vi "Main.vi"() -> ()   [LabVIEW 2022 SP3]
doc: "This template is for the Queued Message Handler design pattern.\n\nThe Event Handling Loop generates messages based on user interface actions.\n\nThe Message Handling Loop processes messages generated by the Event Handling Loop, or by other messages. The messages are string values, so new messages can be added easily to the Message Cases case structure in the Message Handling Loop. Each message cluster can also provide an optional value for Message Data, which is a variant that can be converted to whatever message-specific data is required."
uses:
  controls/UI Data.ctl
  support/Boiler System Globals.vi
  support/Message Queue/Message Queue.lvlib
  support/User Event - Stop/User Event - Stop.lvlib
  Boiler/Boiler.lvlib
panel:
  out "Display <Replace Me>":string
  in  "Do Something Else <Replace Me>":bool
  in  "Do Something <Replace Me>":bool
  in  "Stop Button":bool
  # "These controls have associated \"Value Changed\" events configured in the Event Structure on the diagram.\n\nReplace them (and reconfigure the Event Structure) with the controls you need for your application."
  # "This template is for the Queued Message Handler design pattern.\n\nSee the block diagram for more information on how to use this template."
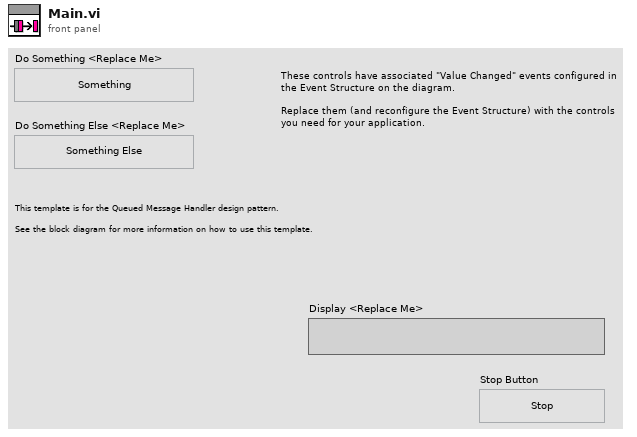
[diagram p1: front panel]
types:
  T1 = typedef "UI Data.ctl" = cluster{"Boolean <Replace Me>":bool, "String <Replace Me>":string, "Numeric <Replace Me>":dbl, "Do Something Ref":refnum<vi>, "Do Something Else Ref":refnum<vi>, "Data Display Ref":refnum<vi>, "Stop Button Ref":refnum<vi>}
  T2 = typedef "Notifiers.ctl" = cluster{"Handshake":refnum<notifier>, "Flame Level":refnum<notifier>, "Controller Exit":refnum<notifier>, "Boiler Ext":refnum<notifier>}
  T3 = typedef "Message Queue.lvlib/All Message Queues.ctl" = cluster{"MHL":refnum<queue>, "Boiler Controller":refnum<queue>, "Boiler":refnum<queue>}
  T4 = enum32{"invalid app kind", "Development System", "Run Time System", "Student Edition", "Embedded LabVIEW", "Evaluation", "Custom"}
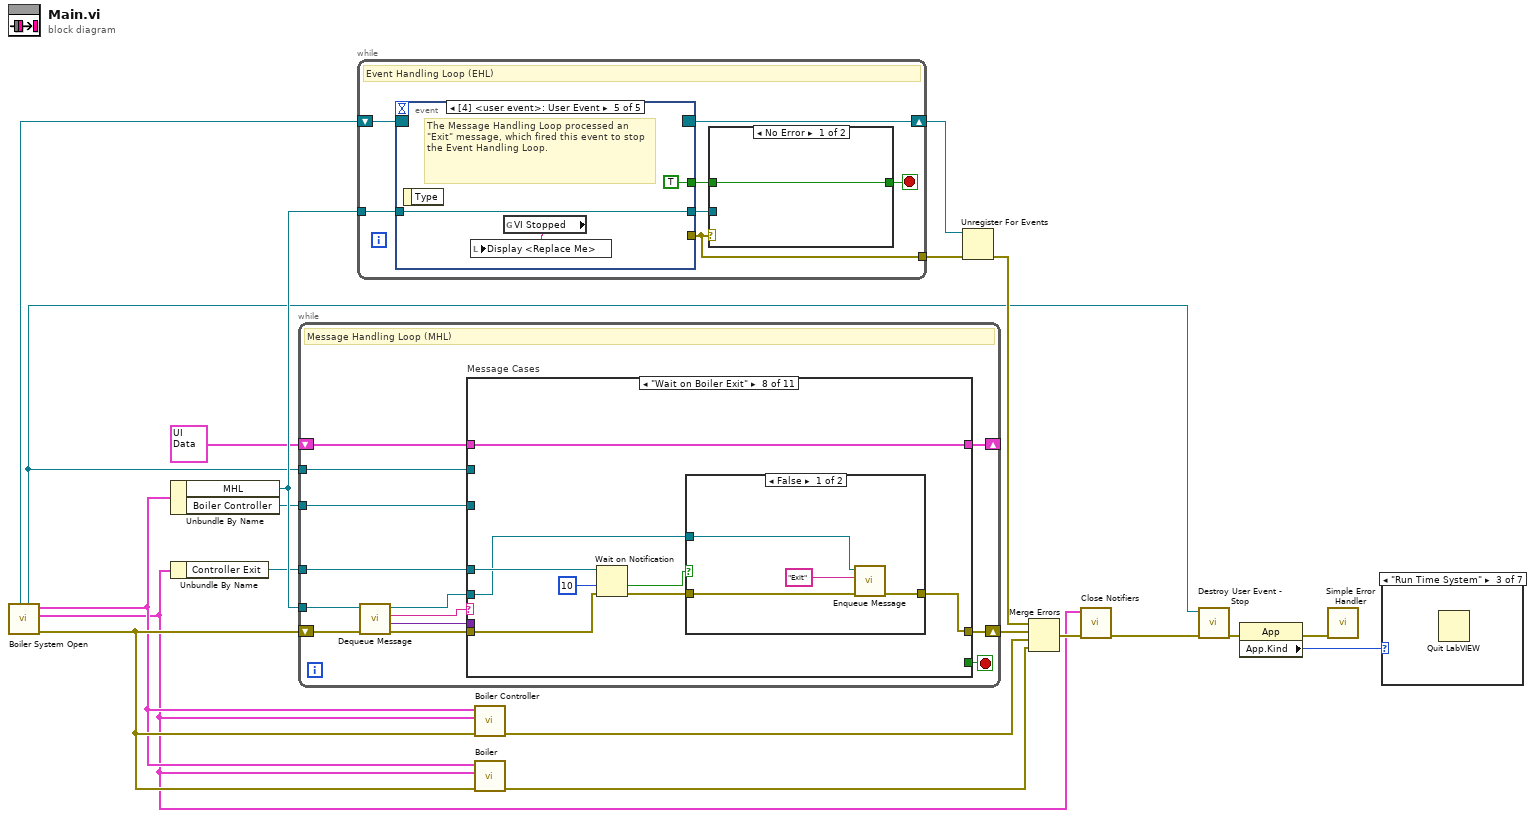
[diagram p0: block diagram]
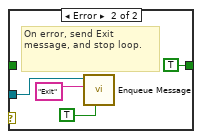
[diagram p8: hidden frame]
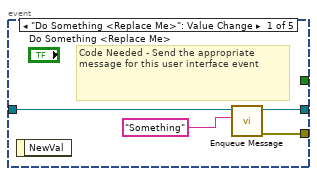
[diagram p9: hidden frame]
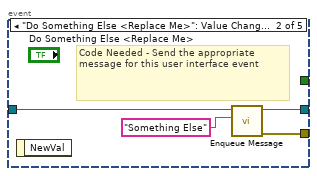
[diagram p10: hidden frame]
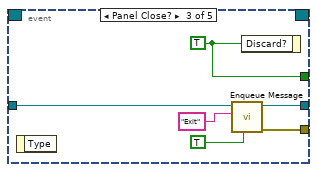
[diagram p11: hidden frame]
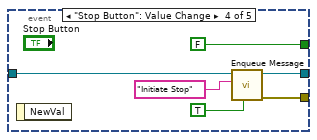
[diagram p12: hidden frame]
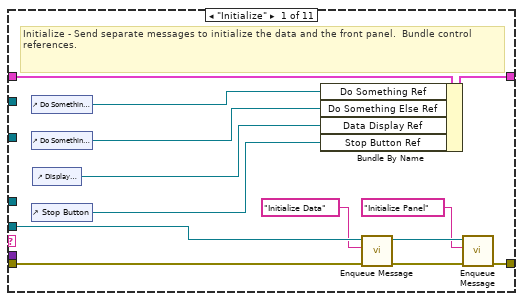
[diagram p13: hidden frame]
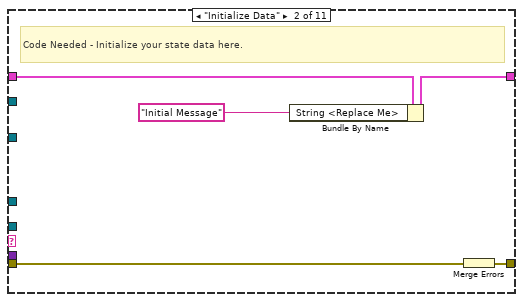
[diagram p14: hidden frame]
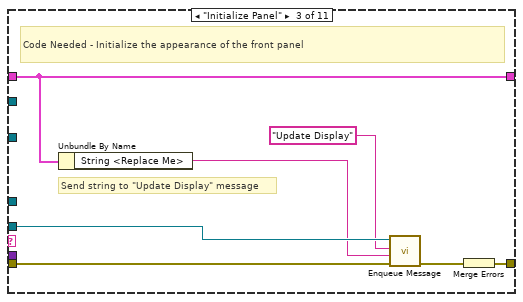
[diagram p15: hidden frame]
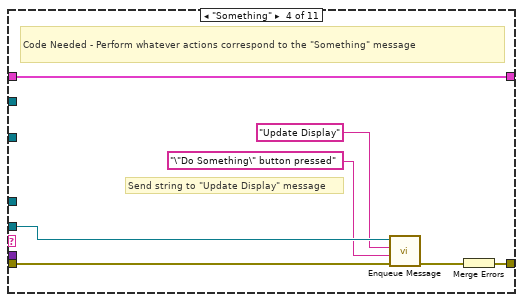
[diagram p16: hidden frame]
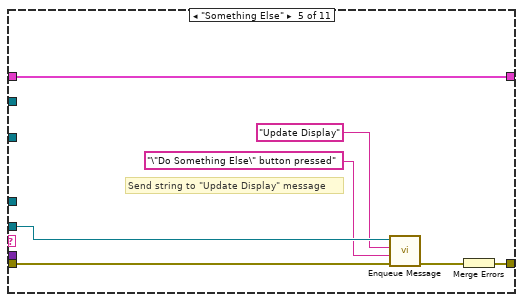
[diagram p17: hidden frame]
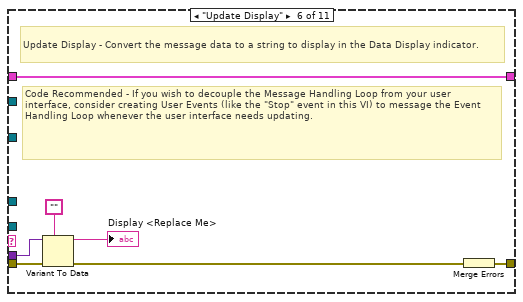
[diagram p18: hidden frame]
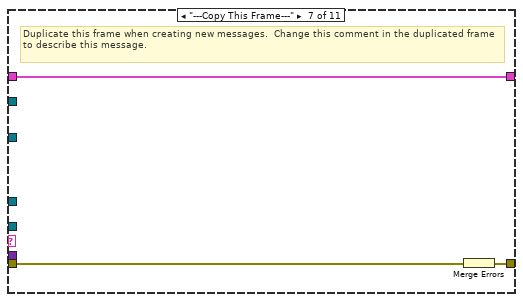
[diagram p19: hidden frame]
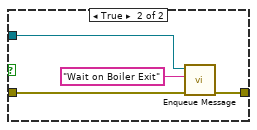
[diagram p20: hidden frame]
diagram:
  n1 = call "Boiler System Open.vi"() -> ("error out"=w7:errorcluster, "Notifiers"=w2:T2, "Message Queues"=w6:T3, "User Event - Stop"=w8:refnum<user-event>, "Stop Event Registration Refnum"=w9:refnum<event-registration>)  [unwired: 7 in]
  n2 = Unbundle By Name(w6) -> ("MHL"=w19:refnum<queue>, "Boiler Controller"=w14:refnum<queue>)
  n3 = Unbundle By Name(w2) -> ("Controller Exit"=w5:refnum<notifier>)
  n4 = while {
    tunnel: w19 -> [w23]
    shift-right: [w32] -> _
    shift-left: T1 {"Boolean <Replace Me>"=TRUE, "String <Replace Me>"="", "Numeric <Replace Me>"=0.0, "Do Something Ref"=refnum, "Do Something Else Ref"=refnum, "Data Display Ref"=refnum, "Stop Button Ref"=refnum} ("Data Cluster") -> [w33]
    tunnel: w8 -> [w29]
    shift-right: [w30] -> w20
    shift-left: w7 -> [w28]
    tunnel: w14 -> [w22]
    tunnel: w5 -> [w21]
    stop <- w31 stop-if-true
    # "Message Handling Loop (MHL)"
    n5 = call "Dequeue Message.vi"("error in"=w28, "Message Queue"=w23) -> ("error out"=w27:errorcluster, "Message Data"=w25:variant, "Message"=w26:string, "dup Message Queue"=w24:refnum<queue>)  [unwired: 6 in]
    n6 = case "Message Cases" shown="\"Wait on Boiler Exit\"" w26 {
      selector: w26 -> [_ _ _ _ _ _ _ _ _ _ w118]
      tunnel: w24 -> [w42 _ w55 w61 w68 _ _ w84 w100 w114 _]
      tunnel: w27 -> [w45 w51 w56 w63 w70 w77 w82 w89 w105 w109 _]
      tunnel: [w46 w47 w57 w64 w71 w78 w80 w83 w103 w110 w116] -> w30
      tunnel: w33 -> [w39 w50 w58 w65 w72 w79 w81 w90 w106 w113 w120]
      tunnel: [w38 w49 w58 w65 w72 w79 w81 w90 w106 w113 w120] -> w32
      tunnel: [_ _ _ _ _ _ _ _ _ TRUE _] -> w31
      tunnel: w25 -> [_ _ _ _ _ w76 _ _ _ _ _]
      tunnel: w29 -> [_ _ _ _ _ _ _ _ _ w108 _]
      tunnel: w22 -> [_ _ _ _ _ _ _ _ w99 _ _]
      tunnel: w21 -> [_ _ _ _ _ _ _ w88 _ _ _]
      frame "Initialize" {
        # "Initialize - Send separate messages to initialize the data and the front panel.  Bundle control references."
        n7 = control-ref of="Do Something <Replace Me>"() -> (w37:refnum<vi>)
        n8 = control-ref of="Do Something Else <Replace Me>"() -> (w36:refnum<vi>)
        n9 = control-ref of="Stop Button"() -> (w34:refnum<vi>)
        n10 = control-ref of="Display <Replace Me>"() -> (w35:refnum<vi>)
        n11 = Bundle By Name(cluster=w39, "Do Something Ref"=w37, "Do Something Else Ref"=w36, "Data Display Ref"=w35, "Stop Button Ref"=w34) -> (w38:T1)
        n12 = call "Enqueue Message.vi"("error in"=w45, "Message"="Initialize Data", "Message Queue"=w42) -> ("error out"=w44:errorcluster, "dup Message Queue"=w43:refnum<queue>)  [unwired: 7 in]
        n13 = call "Enqueue Message.vi"("error in"=w44, "Message"="Initialize Panel", "Message Queue"=w43) -> ("error out"=w46:errorcluster)  [unwired: 7 in, 1 out]
      }
      frame "Initialize Data" {
        # "Code Needed - Initialize your state data here."
        n14 = Bundle By Name(cluster=w50, "String <Replace Me>"="Initial Message" ("Initial Message")) -> (w49:T1)
        n15 = Merge Errors(w51) -> (w47:errorcluster)
      }
      frame "Initialize Panel" {
        # "Send string to \"Update Display\" message"
        # "Code Needed - Initialize the appearance of the front panel"
        n16 = Unbundle By Name(w58) -> ("String <Replace Me>"=w52:string)
        n17 = call "Enqueue Message.vi"("error in"=w56, "Message Data"=w52, "Message"="Update Display", "Message Queue"=w55) -> ("error out"=w54:errorcluster)  [unwired: 6 in, 1 out]
        n18 = Merge Errors(w54) -> (w57:errorcluster)
      }
      frame "Something" {
        # "Send string to \"Update Display\" message"
        # "Code Needed - Perform whatever actions correspond to the \"Something\" message"
        n19 = call "Enqueue Message.vi"("error in"=w63, "Message Data"="\"Do Something\" button pressed" ("\"Do Something\" button pressed"), "Message"="Update Display", "Message Queue"=w61) -> ("error out"=w62:errorcluster)  [unwired: 6 in, 1 out]
        n20 = Merge Errors(w62) -> (w64:errorcluster)
      }
      frame "Something Else" {
        # "Send string to \"Update Display\" message"
        n21 = call "Enqueue Message.vi"("error in"=w70, "Message Data"="\"Do Something Else\" button pressed" ("\"Do Something Else\" button pressed"), "Message"="Update Display", "Message Queue"=w68) -> ("error out"=w69:errorcluster)  [unwired: 6 in, 1 out]
        n22 = Merge Errors(w69) -> (w71:errorcluster)
      }
      frame "Update Display" {
        # "Code Recommended - If you wish to decouple the Message Handling Loop from your user interface, consider creating User Events (like the \"Stop\" event in this VI) to message the Event Handling Loop whenever the user interface needs updating."
        # "Update Display - Convert the message data to a string to display in the Data Display indicator."
        n23 = Variant To Data(error in=w77, type="", Variant=w76) -> (data=→"Display <Replace Me>":string, error out=w74:errorcluster)
        n24 = Merge Errors(w74) -> (w78:errorcluster)
      }
      frame "---Copy This Frame---" {
        # "Duplicate this frame when creating new messages.  Change this comment in the duplicated frame to describe this message."
        n25 = Merge Errors(w82) -> (w80:errorcluster)
      }
      frame "Wait on Boiler Exit" {
        n26 = Wait on Notification(notifier=w88, timeout in ms (-1)=10, error in (no error)=w89) -> (timed out?=w85:bool, error out=w86:errorcluster)  [unwired: 1 in, 2 out]
        n27 = case shown="False" w85 {
          tunnel: w86 -> [w93 w98]
          tunnel: w84 -> [w92 w97]
          tunnel: [w94 w96] -> w83
          frame False {
            n28 = call "Enqueue Message.vi"("error in"=w93, "Message"="Exit", "Message Queue"=w92) -> ("error out"=w94:errorcluster)  [unwired: 7 in, 1 out]
          }
          frame True {
            n29 = call "Enqueue Message.vi"("error in"=w98, "Message"="Wait on Boiler Exit", "Message Queue"=w97) -> ("error out"=w96:errorcluster)  [unwired: 7 in, 1 out]
          }
        }
      }
      frame "Initiate Stop" {
        # "When stopping, first send a message to stop the boiler controller.\nThen wait for the boiler and boiler controller to ext"
        n30 = call "Enqueue Message.vi"("error in"=w105, "Message"="Exit", "Message Queue"=w99) -> ("error out"=w104:errorcluster)  [unwired: 7 in, 1 out]
        n31 = call "Enqueue Message.vi"("error in"=w104, "Message"="Wait on Boiler Exit", "Message Queue"=w100) -> ("error out"=w103:errorcluster)  [unwired: 7 in, 1 out]
      }
      frame "Exit" {
        # "Stop the VI"
        # "Release the message queue reference"
        n32 = call "Fire User Event - Stop.vi"("User Event - Stop"=w108) -> ("error out"=w107:errorcluster)  [unwired: 10 in]
        n33 = Release Queue(queue=w114, error in (no error)=w109) -> (error out=w111:errorcluster)  [unwired: 1 in, 2 out]
        n34 = Merge Errors(w107, w111) -> (w110:errorcluster)
      }
      frame Default {
        # "'Default' case only runs if there is a message that isn't defined in any of the other cases.  Output a programming error."
        n35 = Format Into String(format string="The invalid message string \"%s\" was received in the Message Handling Loop." ("Unknown Message Error Text"), w118) -> (resulting string=w115:string)  [unwired: 2 in, 1 out]
        n36 = call <vilib>:"Error Cluster From Error Code.vi"("error message (\"\")"=w115, "error code (0)"=1) -> ("error out"=w116:errorcluster)  [unwired: 7 in]
      }
    }
  }
  n37 = while {
    tunnel: w19 -> [w127]
    tunnel: [w123] -> w17
    shift-right: [w121] -> w16
    shift-left: w9 -> [w122]
    stop <- w125 stop-if-true
    # "Event Handling Loop (EHL)"
    n38 = event shown="[4] <user event>: User Event" {
      selector: w122 -> [_ _ _ _ _]
      dyn-events: [_ _ _ _ _] -> w121
      timeout: _ -> [_ _ _ _ _]
      tunnel: [_ _ w146 FALSE ("Discard?") TRUE ("Discard?")] -> w126
      tunnel: w127 -> [w136 w140 w145 w152 w155]
      tunnel: [w135 w138 w144 w151 _] -> w123
      tunnel: [w134 w139 w143 w149 w155] -> w124
      event "Do Something <Replace Me>": Value Change {
        # "Code Needed - Send the appropriate message for this user interface event"
        n39 = event-data() -> ()  [unwired: 1 in, 1 out]
        n40 = call "Enqueue Message.vi"("Message"="Something", "Message Queue"=w136) -> ("error out"=w135:errorcluster, "dup Message Queue"=w134:refnum<queue>)  [unwired: 8 in]
      }
      event "Do Something Else <Replace Me>": Value Change {
        # "Code Needed - Send the appropriate message for this user interface event"
        n41 = event-data() -> ()  [unwired: 1 in, 1 out]
        n42 = call "Enqueue Message.vi"("Message"="Something Else", "Message Queue"=w140) -> ("error out"=w138:errorcluster, "dup Message Queue"=w139:refnum<queue>)  [unwired: 8 in]
      }
      event Panel Close? {
        w146 = TRUE ("Discard?")
        n43 = event-data() -> ()  [unwired: 1 in, 1 out]
        n44 = call "Enqueue Message.vi"("Priority Message? (F)"=TRUE, "Message"="Exit", "Message Queue"=w145) -> ("error out"=w144:errorcluster, "dup Message Queue"=w143:refnum<queue>)  [unwired: 7 in]
        n45 = event-data("Discard?"=w146) -> ()  [unwired: 1 in, 1 out]
      }
      event "Stop Button": Value Change {
        n46 = event-data() -> ()  [unwired: 1 in, 1 out]
        n47 = call "Enqueue Message.vi"("Priority Message? (F)"=TRUE, "Message"="Initiate Stop", "Message Queue"=w152) -> ("error out"=w151:errorcluster, "dup Message Queue"=w149:refnum<queue>)  [unwired: 7 in]
      }
      event User Event {
        # "The Message Handling Loop processed an \"Exit\" message, which fired this event to stop the Event Handling Loop."
        n48 = event-data() -> ()  [unwired: 1 in, 1 out]
        n49 = global read "Boiler System Globals.vi" "VI Stopped"() -> (w153:string)
        n50 = local write "Display <Replace Me>"(w153) -> ()
      }
    }
    n51 = case shown="No Error" w123 {
      tunnel: [w128 TRUE ("Discard?")] -> w125
      tunnel: w126 -> [w128 _]
      tunnel: w124 -> [_ w131]
      frame No Error {
      }
      frame Error {
        # "On error, send Exit message, and stop loop."
        n52 = call "Enqueue Message.vi"("Priority Message? (F)"=TRUE, "Message"="Exit", "Message Queue"=w131) -> ()  [unwired: 7 in, 2 out]
      }
    }
  }
  n53 = call "Boiler Controller.vi"("error in"=w7, "Notifiers"=w2, "Message Queues"=w6) -> ("error out"=w13:errorcluster)  [unwired: 8 in]
  n54 = call "Boiler.vi"("error in"=w7, "Notifiers"=w2, "Message Queues"=w6) -> ("error out"=w1:errorcluster)  [unwired: 8 in]
  n55 = Unregister For Events(event registration refnum=w16, error in=w17) -> (error out=w18:errorcluster)
  n56 = Merge Errors(w18, w20, w13, w1) -> (w4:errorcluster)
  n57 = call "Close Notifiers.vi"("error in"=w4, "Notifiers"=w2) -> ("error out"=w3:errorcluster)  [unwired: 9 in]
  n58 = call "Destroy User Event - Stop.vi"("error in"=w3, "User Event - Stop"=w8) -> ("error out"=w12:errorcluster)  [unwired: 9 in]
  n59 = property class="App"(error in=w12) -> (error out=w11:errorcluster, "App.Kind"=w10:T4)  [unwired: 1 in, 1 out]
  n60 = call <vilib>:"Simple Error Handler.vi"("error in (no error)"=w11) -> ()  [unwired: 4 in, 5 out]
  n61 = case shown="\"Run Time System\"" w10 {
    frame "invalid app kind", Default {
    }
    frame "Development System" {
    }
    frame "Run Time System" {
      n62 = Quit LabVIEW() -> ()  [unwired: 1 in]
    }
    frame "Student Edition" {
    }
    frame "Embedded LabVIEW" {
    }
    frame "Evaluation" {
    }
    frame "Custom" {
    }
  }
